vi "Validate Current.vi"(1 "Current Array":T1=[0, 0, 0, 0, 0]) -> (0 "Current Out":u8[](array[numeric]))   [LabVIEW 2019]
uses:
  Controls/Stim Current Array.ctl
panel:
  in  "Current":u8 caption="Current (mA)"
  out "Warning":string
  out "Current":u8 caption="Current (mA)"
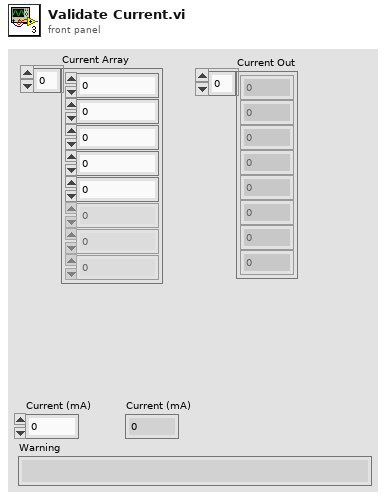
[diagram p1: front panel]
types:
  T1 = typedef "Stim Current Array.ctl" = u8[]
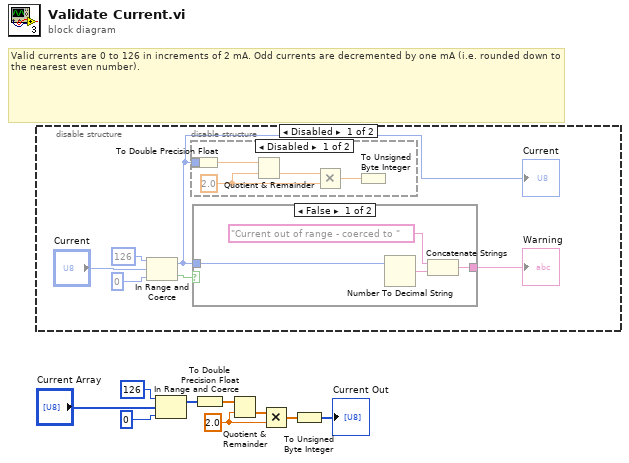
[diagram p0: block diagram]
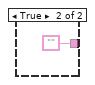
[diagram p3: hidden frame]
diagram:
  w3 = 2.0 ("y")
  # "Valid currents are 0 to 126 in increments of 2 mA. Odd currents are decremented by one mA (i.e. rounded down to the nearest even number)."
  n1 = disable-structure shown="Disabled" {
    frame Disabled {
      n2 = In Range and Coerce(upper limit=u8 126, x="Current", lower limit=u8 0) -> (coerced(x)=w10:u8, In Range?=w13:bool)
      "Current" <- w10
      n3 = disable-structure shown="Disabled" {
        disable-tunnel: w10 -> [w20 _]
        frame Disabled {
          w18 = 2.0 ("y")
          n4 = To Double Precision Float(number=w20) -> (double precision float=w17:dbl)
          n5 = Quotient & Remainder(x=w17, y=w18) -> (floor(x/y)=w19:dbl)  [unwired: 1 out]
          n6 = Multiply(x=w19, y=w18) -> (x*y=w21:dbl)
          n7 = To Unsigned Byte Integer(number=w21) -> (unsigned 8bit integer=w16:u8)
        }
        frame Enabled {
        }
      }
      n8 = case shown="False" w13 {
        tunnel: w10 -> [w22 _]
        tunnel: [w23 ""] -> w14
        frame False {
          n9 = Number To Decimal String(number=w22) -> (decimal integer string=w24:string)  [unwired: 1 in]
          n10 = Concatenate Strings("Current out of range - coerced to ", w24) -> (w23:string)
        }
        frame True {
        }
      }
      "Warning" <- w14
    }
    frame Enabled {
    }
  }
  n11 = In Range and Coerce(upper limit=u8 126, x="Current Array", lower limit=u8 0) -> (coerced(x)=w6:u8[])  [unwired: 1 out]
  n12 = To Double Precision Float(number=w6) -> (double precision float=w5:dbl[])
  n13 = Quotient & Remainder(x=w5, y=w3) -> (floor(x/y)=w4:dbl[])  [unwired: 1 out]
  n14 = Multiply(x=w4, y=w3) -> (x*y=w2:dbl[])
  n15 = To Unsigned Byte Integer(number=w2) -> (unsigned 8bit integer=→"Current Out":u8[])
